vi "Create Pattern Script(Data_3W).vi"(7 "DataType":T1, 8 "error in (no error)":errorcluster, 11 "Data":u16 format="%x") -> (0 "error out":errorcluster, 3 "String":string)   [LabVIEW 2018, in "SPI_Frame_Root.lvclass"]
uses:
  SPI_Frame_Root.lvclass
  DataType.ctl
  Classes/BML_Frame_Root/BML_Frame_Root.lvclass
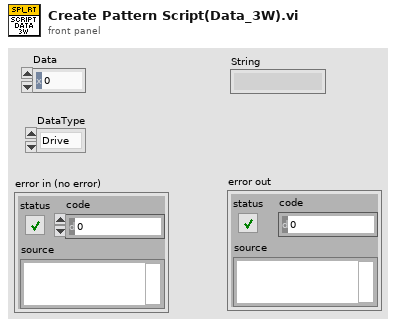
[diagram p1: front panel]
types:
  T1 = typedef "SPI_Frame_Root.lvclass/DataType.ctl" = enum16{"Drive", "Compare", "Read"}
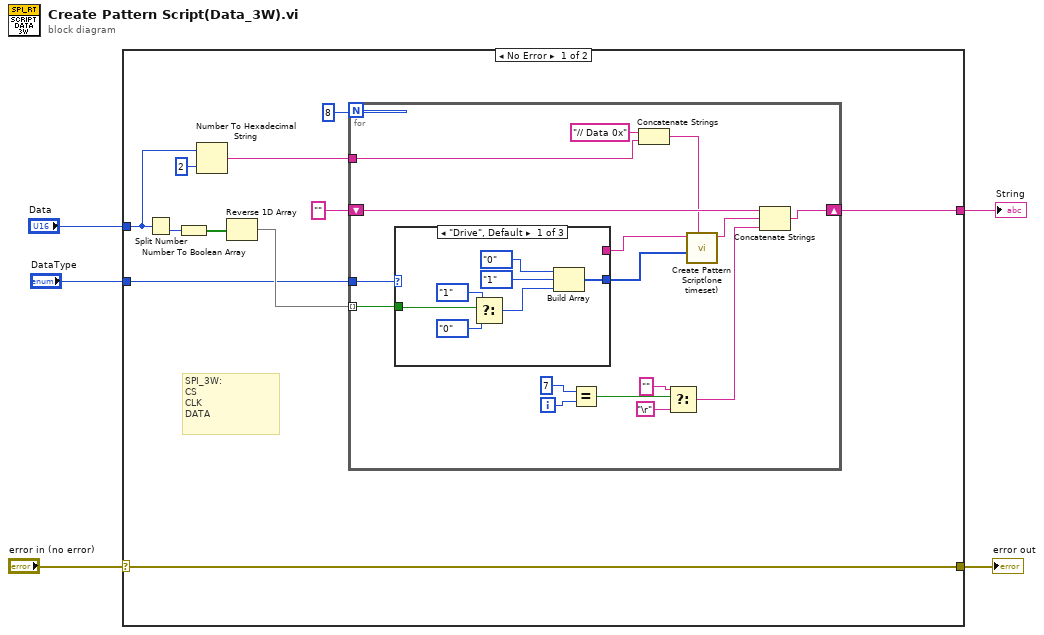
[diagram p0: block diagram]
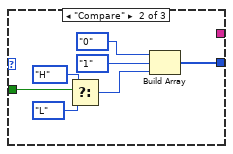
[diagram p2: hidden frame]
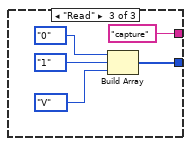
[diagram p3: hidden frame]
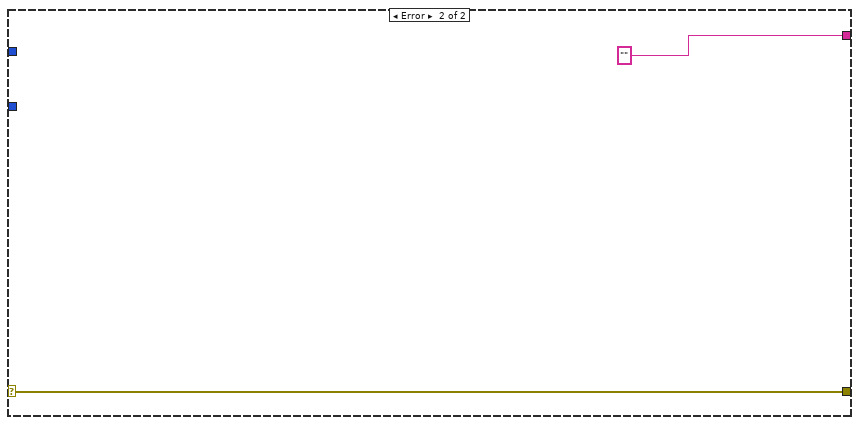
[diagram p4: hidden frame]
diagram:
  n1 = case shown="No Error" "error in (no error)" {
    selector: "error in (no error)" -> [w16 w52]
    tunnel: [w8 ""] -> w4
    tunnel: [w16 w52] -> w3
    tunnel: "Data" -> [w7 _]
    tunnel: "DataType" -> [w9 _]
    frame No Error {
      # "SPI_3W:\nCS\nCLK\nDATA"
      n2 = Split Number(x=w7) -> (lo(x)=w6:u8)  [unwired: 1 out]
      n3 = Number To Boolean Array(number=w6) -> (Boolean array=w12:bool[])
      n4 = Number To Hexadecimal String(1:i16 2 ("width (-)"), 2:w7) -> (0:w13:string)
      n5 = Reverse 1D Array(array=w12) -> (reversed array=w10:bool[])
      n6 = for {
        N: 8 -> [_]
        shift-right: [w27] -> w8
        shift-left: "" -> [w26]
        tunnel: w13 -> [w22]
        tunnel: w10 -> [w19] mode=indexing
        tunnel: w9 -> [w20]
        i -> [w32]
        n7 = case shown="\"Drive\", Default" w20 {
          tunnel: w19 -> [w36 w44 _]
          tunnel: [w35 w42 w50] -> w18
          tunnel: [_ _ "capture" ("opcode")] -> w17
          frame "Drive", Default {
            n8 = Select(t=enum16{"0", "1", "L", "H", "X", "V", "D", "M"}."1" ("PinState"), s=w36, f=enum16{"0", "1", "L", "H", "X", "V", "D", "M"}."0") -> (s? t:f=w33:enum16{"0", "1", "L", "H", "X", "V", "D", "M"})
            n9 = Build Array(enum16{"0", "1", "L", "H", "X", "V", "D", "M"}."0" ("PinState"), enum16{"0", "1", "L", "H", "X", "V", "D", "M"}."1" ("element"), w33) -> (w35:enum16{"0", "1", "L", "H", "X", "V", "D", "M"}[])
          }
          frame "Compare" {
            n10 = Select(t=enum16{"0", "1", "L", "H", "X", "V", "D", "M"}."H" ("PinState"), s=w44, f=enum16{"0", "1", "L", "H", "X", "V", "D", "M"}."L") -> (s? t:f=w40:enum16{"0", "1", "L", "H", "X", "V", "D", "M"})
            n11 = Build Array(enum16{"0", "1", "L", "H", "X", "V", "D", "M"}."0" ("PinState"), enum16{"0", "1", "L", "H", "X", "V", "D", "M"}."1" ("element"), w40) -> (w42:enum16{"0", "1", "L", "H", "X", "V", "D", "M"}[])
          }
          frame "Read" {
            n12 = Build Array(enum16{"0", "1", "L", "H", "X", "V", "D", "M"}."0" ("PinState"), enum16{"0", "1", "L", "H", "X", "V", "D", "M"}."1" ("element"), enum16{"0", "1", "L", "H", "X", "V", "D", "M"}."V" ("element")) -> (w50:enum16{"0", "1", "L", "H", "X", "V", "D", "M"}[])
          }
        }
        n13 = Equal?(x=7, y=w32) -> (x = y?=w30:bool)
        n14 = Concatenate Strings("// Data 0x" ("string"), w22) -> (w21:string)
        n15 = Select(t="", s=w30, f="\r") -> (s? t:f=w25:string)
        n16 = call "Create Pattern Script(one timeset).vi"("Notes"=w21, "PinState"=w18, "opcode"=w17) -> ("string out"=w24:string)  [unwired: 8 in]
        n17 = Concatenate Strings(w26, w24, w25) -> (w27:string)
      }
    }
    frame Error {
    }
  }
  "String" <- w4
  "error out" <- w3
